vi "API_Key.vi"() -> ()   [LabVIEW 2024]
panel:
  out "API_Key":string
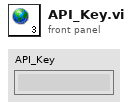
[diagram p1: front panel]
diagram:
